vi "WayPointFollowing.vi"() -> ()   [LabVIEW 2010]
uses:
  5.0-Global.vi
  <vilib>/Analysis/1siggen.llb/Ramp Pattern by Samples.vi
  <vilib>/gmath/statdist.llb/Normal PDF.vi
  <vilib>/gmath/NI_Gmath.lvlib
  <vilib>/Analysis/NI_AALBase.lvlib
panel:
  out "Where-to-Where In Indicator":T1(array[cluster])
  out "ActCommand":dbl[](array[numeric])
  in  "InhibitIn":bool
  in  "SupressIn":dbl=1.0
  out "SupressOut":dbl
  out "InhibitOut":bool
  out "Vel":dbl
  out "SteerAngle":dbl
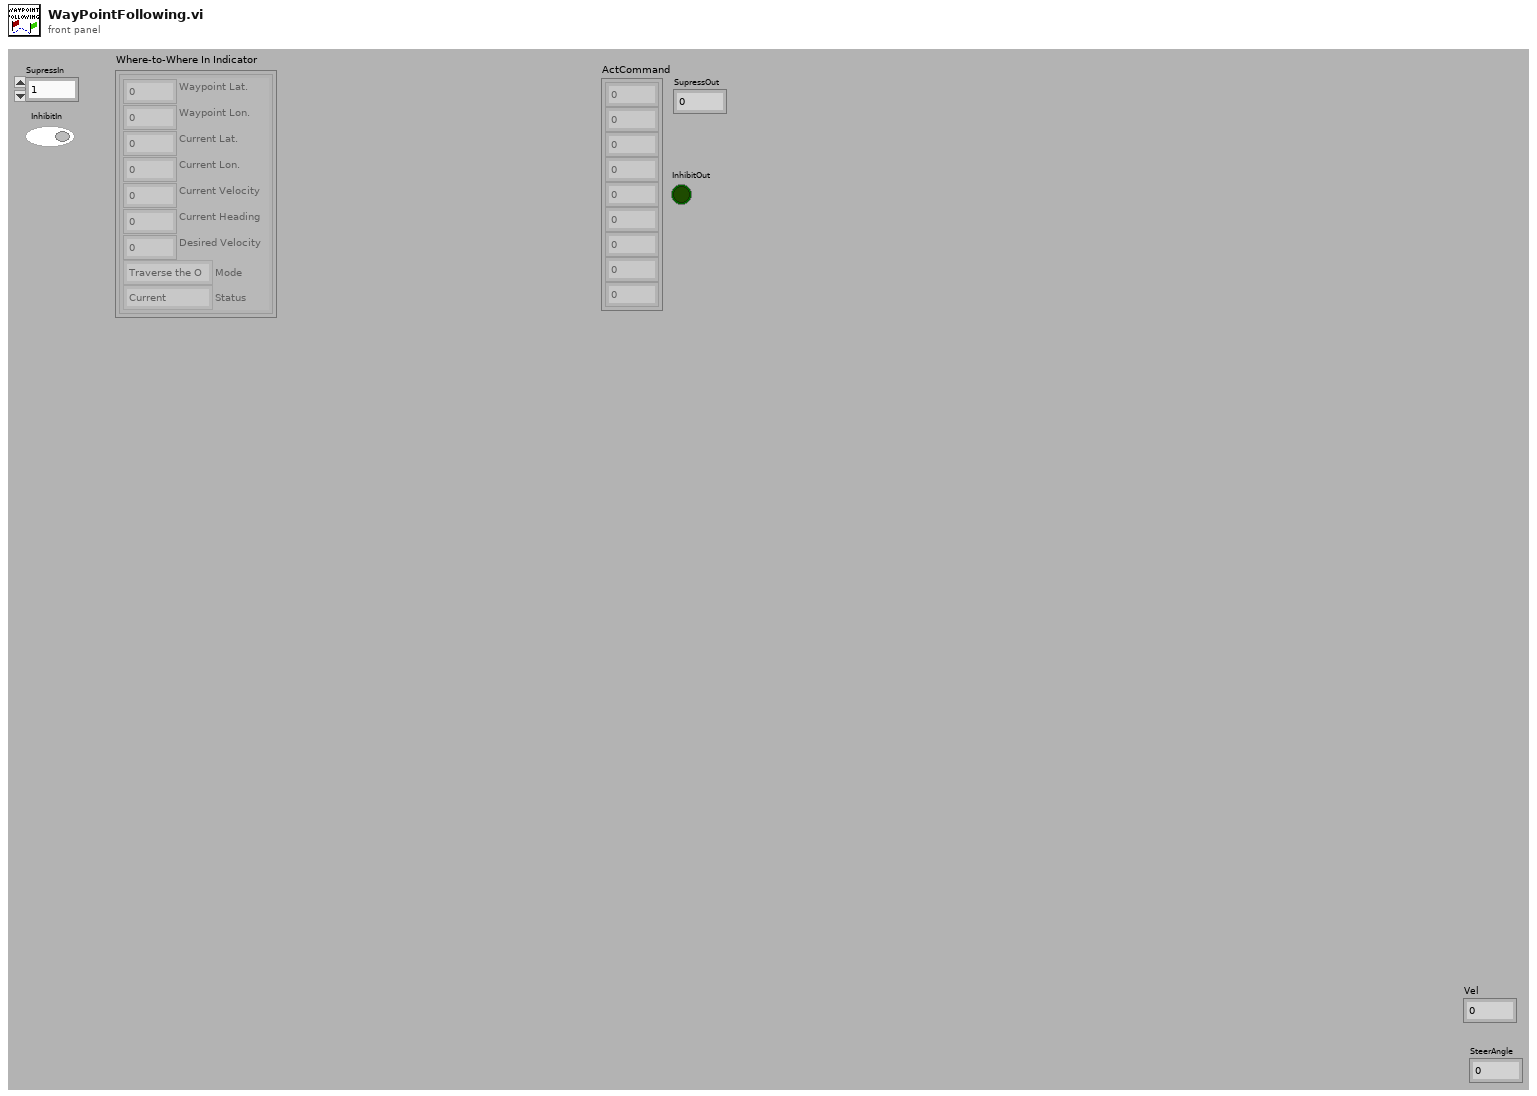
[diagram p1: front panel]
types:
  T1 = cluster{"Waypoint Lat.":dbl, "Waypoint Lon.":dbl, "Current Lat.":dbl, "Current Lon. ":dbl, "Current Velocity":dbl, "Current Heading":dbl, "Desired Velocity":dbl, "Mode":enum16{"Traverse the O"}, "Status":enum16{"Current", "Future", "Past"}}[]
  T2 = cluster{"X (Current)":dbl, "Y (Current) ":dbl, "Heading":dbl, "Steering Angle":dbl}
  T3 = typedef "MDFArray.ctl" = T4[]
  T4 = typedef "MDF Waypoint.ctl" = cluster{"Waypoint #":dbl, "X (waypoint)":ext, "Y (waypoint)":ext, "Vel (desired)":dbl, "Dwell Time":dbl, "Behavior":enum16{"OpenFieldTransit", "WallFollow", "LaneFollow", "ManualMode"}, "Expand1":dbl, "Expand2":dbl, "Expand3":dbl}
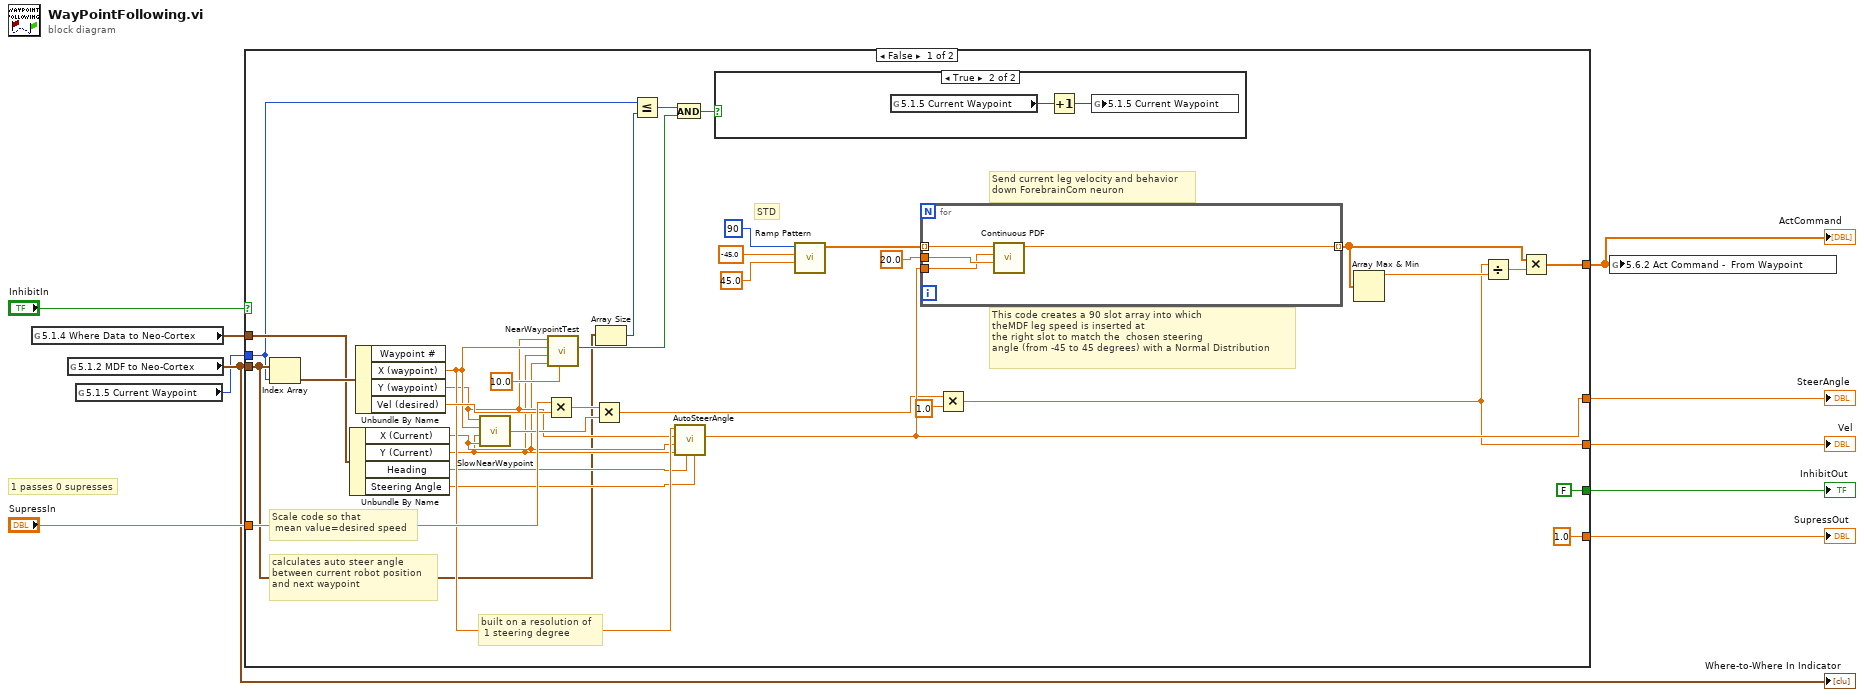
[diagram p0: block diagram]
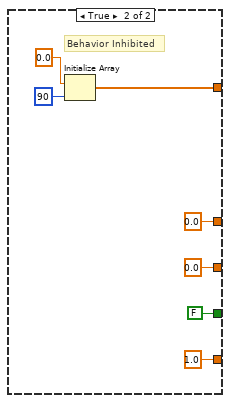
[diagram p3: hidden frame]
diagram:
  # "1 passes 0 supresses"
  n1 = global read "5.0-Global.vi" "5.1.4 Where Data to Neo-Cortex"() -> (w2:T2)
  n2 = global read "5.0-Global.vi" "5.1.2 MDF to Neo-Cortex"() -> (w4:T3)
  "Where-to-Where In Indicator" <- w4
  n3 = global read "5.0-Global.vi" "5.1.5 Current Waypoint"() -> (w1:i32)
  n4 = case shown="False" "InhibitIn" {
    tunnel: "SupressIn" -> [w32 _]
    tunnel: [w34 w55] -> w3
    tunnel: [1.0 ("SupressOut") 1.0 ("SupressOut")] -> w7
    tunnel: [FALSE ("InhibitOut") FALSE ("InhibitOut")] -> w8
    tunnel: w4 -> [w15 _]
    tunnel: [w28 0.0 ("Vel")] -> w9
    tunnel: [w33 0.0 ("SteerAngle")] -> w10
    tunnel: w2 -> [w27 _]
    tunnel: w1 -> [w13 _]
    frame False {
      # "calculates auto steer angle\nbetween current robot position\nand next waypoint"
      # "built on a resolution of\n 1 steering degree"
      # "Scale code so that\n mean value=desired speed"
      # "STD"
      # "This code creates a 90 slot array into which\ntheMDF leg speed is inserted at\nthe right slot to match the  chosen steering\nangle (from -45 to 45 degrees) with a Normal Distribution"
      # "Send current leg velocity and behavior\ndown ForebrainCom neuron"
      n5 = Index Array "Index Array"(array=w15, index=w13) -> (element=w29:T4)
      n6 = Unbundle By Name(w27) -> ("X (Current)"=w19:dbl, "Y (Current)"=w18:dbl, "Heading"=w17:dbl, "Steering Angle"=w16:dbl)
      n7 = Unbundle By Name(w29) -> ("X (waypoint)"=w21:ext, "Y (waypoint)"=w20:ext, "Vel (desired)"=w25:dbl)  [unwired: 1 out]
      n8 = call "SlowNearWaypoint.vi"("X (Current)"=w19, "Y (Current)"=w18, "X (Waypoint)"=w21, "Y (Waypoint)"=w20) -> ("SpeedDecrease"=w23:dbl)  [unwired: 2 in]
      n9 = Multiply(x=w32, y=w25) -> (x*y=w31:dbl)
      n10 = call "NearWaypointTest.vi"("Capture Radius"=10.0, "X (Current)"=w19, "Y (Current)"=w18, "X (Waypoint)"=w21, "Y (Waypoint)"=w20) -> ("AtWaypoint"=w22:bool)  [unwired: 6 in]
      n11 = Multiply(x=w31, y=w23) -> (x*y=w24:dbl)
      n12 = Array Size(array=w15) -> (size(s)=w14:i32)
      n13 = Less Or Equal?(x=w13, y=w14) -> (x <= y?=w11:bool)
      n14 = And(x=w11, y=w22) -> (x .and. y?=w12:bool)
      n15 = call "AutoSteerAngle.vi"("CurrentSteerAngle"=w16, "CurrentDirection"=w17, "Y (Current)"=w18, "X(Current)"=w19, "Y (Waypoint)"=w20, "X (Waypoint)"=w21) -> ("NewSteerAngle"=w33:dbl)  [unwired: 5 in]
      n16 = case shown="True" w12 {
        frame False {
        }
        frame True {
          n17 = global read "5.0-Global.vi" "5.1.5 Current Waypoint"() -> (w46:i32)
          n18 = Increment(x=w46) -> (x+1=w45:i32)
          n19 = global write "5.0-Global.vi" "5.1.5 Current Waypoint"(w45) -> ()
        }
      }
      n20 = call-poly <vilib>:"Ramp Pattern.vi"("start"=45.0, "end"=-45.0 ("end (Normal)"), "samples"=90) -> ("Ramp Pattern"=w37:dbl[])  [unwired: 7 in, 1 out]
      n21 = for {
        tunnel: w37 -> [w50] mode=indexing
        tunnel: 20.0 ("std (Normal)") -> [w49]
        tunnel: [w48] -> w41 mode=indexing
        tunnel: w33 -> [w47]
        n22 = call-poly <vilib>:"Continuous PDF.vi"("std"=w49, "mean"=w47, "x"=w50) -> ("pdf(x)"=w48:dbl)  [unwired: 7 in, 1 out]
      }
      n23 = Multiply(x=w24, y=1.0) -> (x*y=w28:dbl)
      n24 = Array Max & Min(array=w41) -> (max value=w39:dbl)  [unwired: 3 out]
      n25 = Divide(x=w28, y=w39) -> (x/y=w40:dbl)
      n26 = Multiply(x=w41, y=w40) -> (x*y=w34:dbl[])
    }
    frame True {
      # "Behavior Inhibited"
      n27 = Initialize Array "Initialize Array"(0.0 ("element"), 90 ("dimension size")) -> (w55:dbl[])
    }
  }
  "ActCommand" <- w3
  "SupressOut" <- w7
  "InhibitOut" <- w8
  "Vel" <- w9
  "SteerAngle" <- w10
  n28 = global write "5.0-Global.vi" "5.6.2 Act Command -  From Waypoint"(w3) -> ()
